vi "ErrorFlattener.vi"(11 "ErrorIn":i32[](array[numeric])) -> (3 "ErrorReduced":i32[](array[numeric]))   [LabVIEW 2022 SP3]
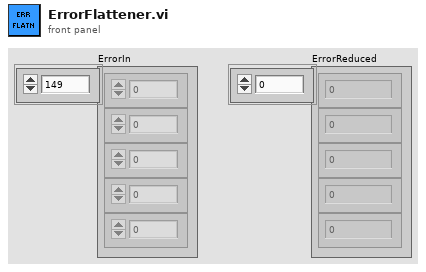
[diagram p1: front panel]
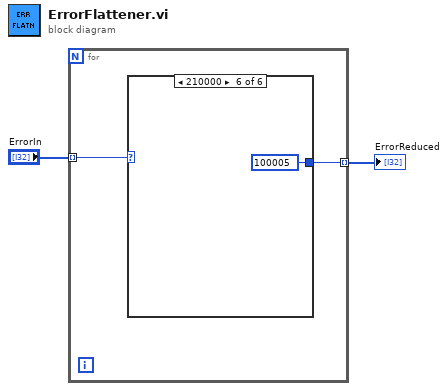
[diagram p0: block diagram]
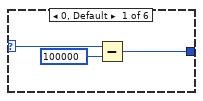
[diagram p2: hidden frame]
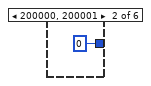
[diagram p3: hidden frame]
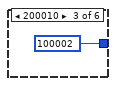
[diagram p4: hidden frame]
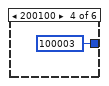
[diagram p5: hidden frame]
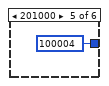
[diagram p6: hidden frame]
diagram:
  n1 = for {
    tunnel: "ErrorIn" -> [w4] mode=indexing
    tunnel: [w3] -> w1 mode=indexing
    n2 = case shown="210000" w4 {
      selector: w4 -> [w7 _ _ _ _ _]
      tunnel: [w5 0 100002 100003 100004 100005] -> w3
      frame 0, Default {
        n3 = Subtract(x=w7, y=100000) -> (x-y=w5:i32)
      }
      frame 200000, 200001 {
      }
      frame 200010 {
      }
      frame 200100 {
      }
      frame 201000 {
      }
      frame 210000 {
      }
    }
  }
  "ErrorReduced" <- w1
